vi "WPI_DMAAddChannelToStream_Gyro.vi"(7 "GyroDeviceRef":T1={"DevStatus"={"status"=FALSE, "code"=0, "source"=""}, "Analog Channel"=enum."AI 1", "Gain (VoltsPerDegree/Second)"=0.0, "Gyro Type"=enum."Analog", "Handle"=0, "SPI Bus"=enum."Invalid", "Device Found"=FALSE, "Sample Rate"=1.0, "Calibrate On Open"=FALSE, "Offset"=0.0} {"Sample Rate" min=0.25 max=100.0 step=0.25}, 8 "error in (no error)":errorcluster, 10 "Gyro Type":T4, 11 "DMARef":T5) -> (0 "error out":errorcluster, 3 "DMARef":T5)   [LabVIEW 2017]
doc: "Specifies the data transferred in the DMA stream. Wire a device reference from the other WPI Robotics Library Open VIs to specify the data you want to receive. The order that the AddChannel VIs add data to the DMA stream defines the order that the Read VI returns the data.\n\nSpecifies the gyro data transferred in the DMA stream.\n\nYou must open a reference to a DMA stream with the Open VI before using this VI.\n\nThis software is licensed. Open the labview\\readme\\WPI Robotics Library Open Source License.txt file for more information."
uses:
  <vilib>/Rock Robotics/WPI/DMA/WPI_DMARef.ctl
  <vilib>/Rock Robotics/WPI/DMA/WPI_DMAGyroType.ctl
  <vilib>/Rock Robotics/WPI/Gyro/WPI_GyroDevRef.ctl
  <vilib>/Rock Robotics/SystemInterfaces/AI/FPGA_AIChannel.ctl
  <vilib>/Rock Robotics/SystemInterfaces/spilib/spi_bus.ctl
  <vilib>/Rock Robotics/WPI/DMA/WPI_DMAChannelTypeEnum.ctl
panel:
  # "Analog"
  # "XRS"
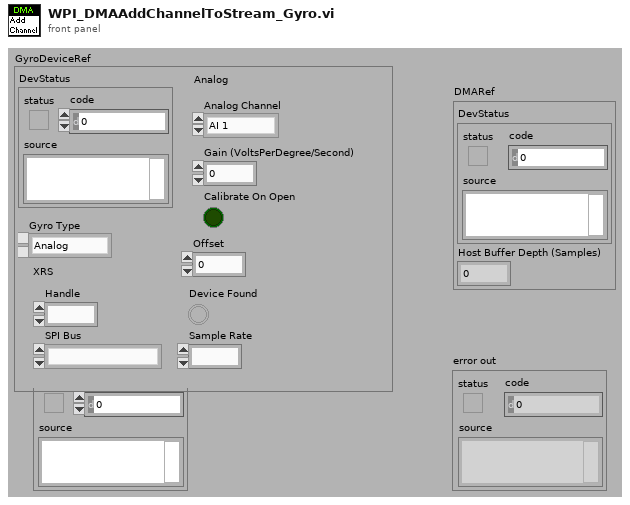
[diagram p1: front panel]
types:
  T1 = typedef "WPI_GyroDevRef.ctl" = cluster{"DevStatus":errorcluster, "Analog Channel":T2, "Gain (VoltsPerDegree/Second)":dbl, "Gyro Type":enum16{"Analog", "XRS450"}, "Handle":i32, "SPI Bus":T3, "Device Found":bool, "Sample Rate":dbl, "Calibrate On Open":bool, "Offset":dbl}
  T2 = typedef "FPGA_AIChannel.ctl" = enum8{"AI 0", "AI 1", "AI 2", "AI 3", "AI MXP 0", "AI MXP 1", "AI MXP 2", "AI MXP 3", "Invalid"}
  T3 = typedef "spi_bus.ctl" = enum16{"SPI On-Board, CS0", "SPI On-Board, CS1", "SPI On-Board, CS2", "SPI On-Board, CS3", "SPI MXP", "Invalid"}
  T4 = typedef "WPI_DMAGyroType.ctl" = enum16{"Angle", "Angular Rate"}
  T5 = typedef "WPI_DMARef.ctl" = cluster{"DevStatus":errorcluster, "Host Buffer Depth (Samples)":u32}
  T6 = typedef "WPI_DMAChannelTypeEnum.ctl" = enum16{"AI (Raw)", "AI (Avg)", "Accumulator", "DI (Raw) Onboard", "DI (Filtered) Onboard", "DI (Raw) MXP", "DI (Filtered) MXP", "Analog Trigger", "Counter", "Counter (Timer)", "Encoder", "Encoder (Timer)", "Time Stamp"}
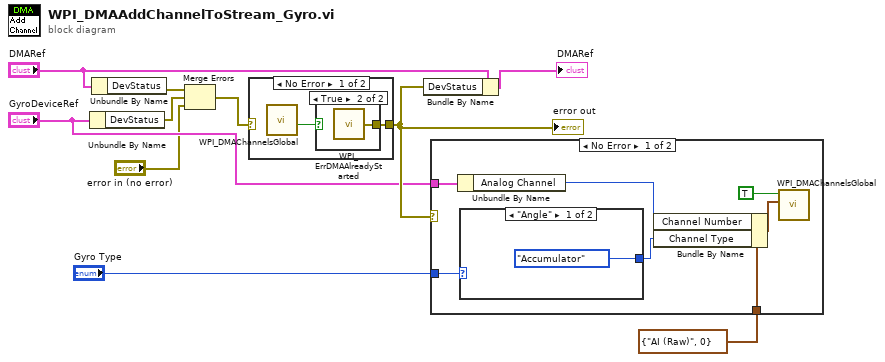
[diagram p0: block diagram]
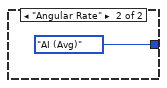
[diagram p2: hidden frame]
diagram:
  n1 = Unbundle By Name("GyroDeviceRef") -> ("DevStatus"=w3:errorcluster)
  n2 = Unbundle By Name("DMARef") -> ("DevStatus"=w4:errorcluster)
  n3 = Merge Errors(w4, w3, "error in (no error)") -> (w1:errorcluster)
  n4 = case shown="No Error" w1 {
    selector: w1 -> [_ w14]
    tunnel: [w11 w14] -> w9
    frame No Error {
      n5 = call <vilib>:"WPI_DMAChannelsGlobal.vi"() -> ("Started"=w12:bool)  [unwired: 4 in, 7 out]
      n6 = case shown="True" w12 {
        tunnel: [_ w13] -> w11
        frame False {
        }
        frame True {
          n7 = call <vilib>:"WPI_ErrDMAAlreadyStarted.vi"() -> ("error out"=w13:errorcluster)
        }
      }
    }
    frame Error {
    }
  }
  "error out" <- w9
  n8 = Bundle By Name(cluster="DMARef", "DevStatus"=w9) -> (→"DMARef":T5)
  n9 = case shown="No Error" w9 {
    tunnel: "GyroDeviceRef" -> [w20 _]
    tunnel: cluster{"Channel Type":T6, "Channel Number":u8} {"Channel Type"=enum."AI (Raw)", "Channel Number"=0} ("Channel") -> [w19 _]
    tunnel: "Gyro Type" -> [w15 _]
    frame No Error {
      n10 = Unbundle By Name(w20) -> ("Analog Channel"=w16:T2)
      n11 = case shown="\"Angle\"" w15 {
        tunnel: [WPI_DMAChannelTypeEnum."Accumulator" ("Channel Type") WPI_DMAChannelTypeEnum."AI (Avg)" ("Channel Type")] -> w17
        frame "Angle" {
        }
        frame "Angular Rate" {
        }
      }
      n12 = Bundle By Name(cluster=w19, "Channel Number"=w16, "Channel Type"=w17) -> (w18:cluster{"Channel Type":T6, "Channel Number":u8})
      n13 = call <vilib>:"WPI_DMAChannelsGlobal.vi"("Channel"=w18, "Add"=TRUE) -> ()  [unwired: 2 in, 8 out]
    }
    frame Error {
    }
  }
